vi "_MPI_CALC.vi"(9 "ofset (mm)":dbl, 10 "IF（GHｚ）":dbl, 11 "LO（GHｚ）":dbl) -> (0 "PU (mag)":dbl, 1 "PL (lmag)":dbl, 3 "SSB_pos(mm)":dbl)   [LabVIEW 2017]
panel:
  out "XYグラフ":cluster{dbl[], dbl[]}(graph)
  in  "MPI_POS(mm)":dbl
  out "SBR (dB)":dbl
  out "n＿LSB":dbl
  out "SSBにするときのMPI間隔":dbl
  out "n＿USB":dbl
  out "λ_LSB":dbl
  out "F_LSB":dbl
  out "λ_USB":dbl
  out "F_USB":dbl
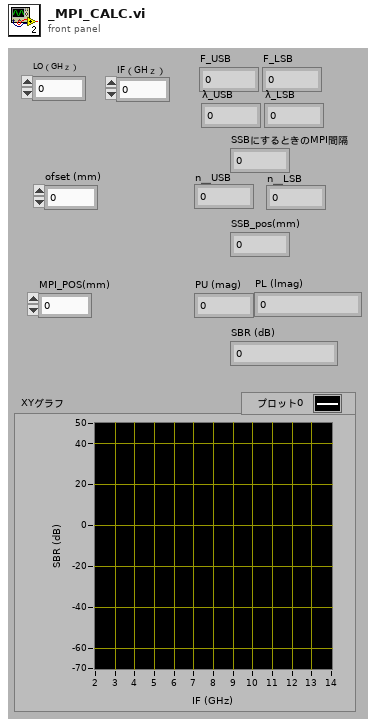
[diagram p1: front panel]
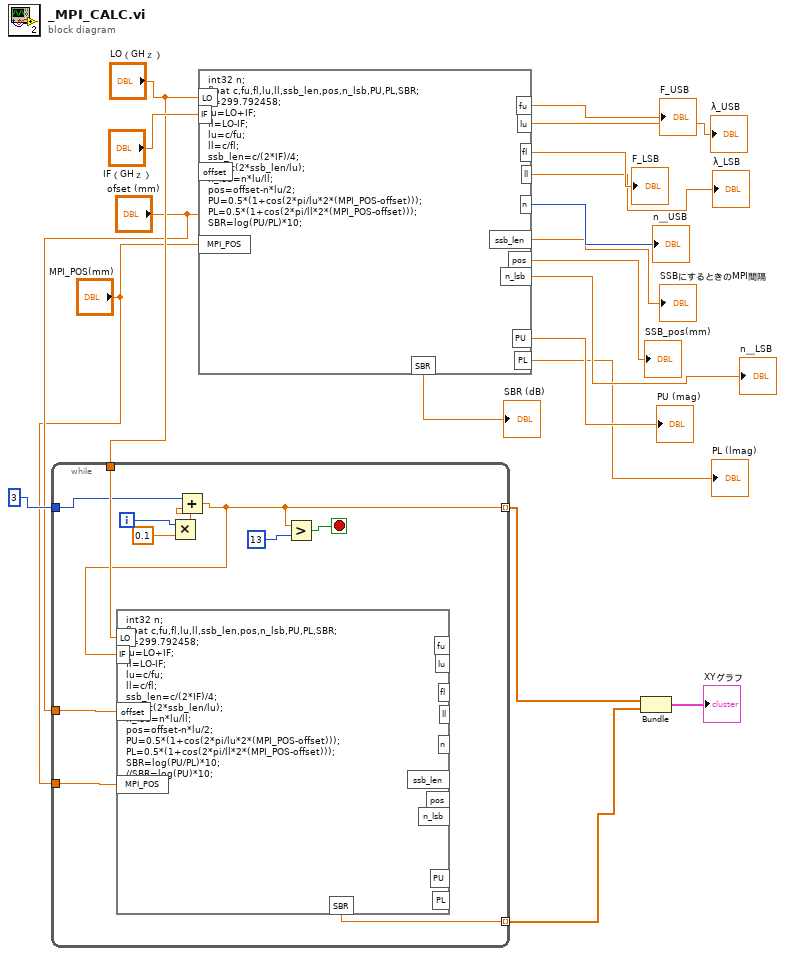
[diagram p0: block diagram]
diagram:
  n1 = while {
    tunnel: "LO（GHｚ）" -> [w28]
    tunnel: "ofset (mm)" -> [w27]
    tunnel: "MPI_POS(mm)" -> [w26]
    tunnel: [w25] -> w3 mode=indexing
    tunnel: 3 -> [w21]
    tunnel: [w20] -> w2 mode=indexing
    i -> [w23]
    stop <- w29 stop-if-true
    n2 = Multiply(x=w23, y=0.1) -> (x*y=w22:dbl)
    n3 = Add(x=w21, y=w22) -> (x+y=w20:dbl)
    n4 = formula code="int32 n;\nfloat c,fu,fl,lu,ll,ssb_len,pos,n_lsb,PU,PL,SBR;\nc=299.792458;\nfu=LO+IF;\nfl=LO-IF;\nlu=c/fu;\nll=c/fl;\nssb_len=c/(2*IF)/4;\nn=int(2*ssb_len/lu);\nn_lsb=n*lu/ll;\npos=offset-n*lu/2;\nPU=0.5*(1+cos(2*pi/lu*2*(MPI_POS-offset)));\nPL=0.5*(1+cos(2*pi/ll*2*(MPI_POS-offset)));\nSBR=log(PU/PL)*10;\n//SBR=log(PU)*10;"("LO"=w28, "IF"=w20, "offset"=w27, "MPI_POS"=w26) -> ("SBR"=w25:dbl)  [unwired: 10 out]
    n5 = Greater?(x=w20, y=13) -> (0:w29:bool)
  }
  n6 = formula code="int32 n;\nfloat c,fu,fl,lu,ll,ssb_len,pos,n_lsb,PU,PL,SBR;\nc=299.792458;\nfu=LO+IF;\nfl=LO-IF;\nlu=c/fu;\nll=c/fl;\nssb_len=c/(2*IF)/4;\nn=int(2*ssb_len/lu);\nn_lsb=n*lu/ll;\npos=offset-n*lu/2;\nPU=0.5*(1+cos(2*pi/lu*2*(MPI_POS-offset)));\nPL=0.5*(1+cos(2*pi/ll*2*(MPI_POS-offset)));\nSBR=log(PU/PL)*10;"("LO"="LO（GHｚ）", "IF"="IF（GHｚ）", "offset"="ofset (mm)", "MPI_POS"="MPI_POS(mm)") -> ("fu"=→"F_USB":dbl, "lu"=→"λ_USB":dbl, "fl"=→"F_LSB":dbl, "ll"=→"λ_LSB":dbl, "n"=→"n＿USB":i32, "ssb_len"=→"SSBにするときのMPI間隔":dbl, "pos"=→"SSB_pos(mm)":dbl, "n_lsb"=→"n＿LSB":dbl, "PU"=→"PU (mag)":dbl, "PL"=→"PL (lmag)":dbl, "SBR"=→"SBR (dB)":dbl)
  n7 = Bundle(w2, w3) -> (→"XYグラフ":cluster{dbl[], dbl[]})  [unwired: 1 in]
